vi "Spi Master.vi"(0 "spi input":T1, 5 "manual assert chip select":bool, 7 "start strobe":bool, 9 "data to write":u64 format="%.0x", 11 "MOSI output enable done":bool=TRUE, 13 "spi transfer settings":T2 {"Direction Change Bit" max=64 step=1; "Transfer Length (bits)" min=1 max=64 step=1}) -> (4 "spi output":T3, 8 "read data valid":bool, 10 "read data":u64 format="%.0x", 14 "ready for input":bool)   [LabVIEW 2014, in "NI SPI IP (FPGA).lvlib"]
doc: "This VI implements a SPI master that is compliant with both 4-wire (unidirectional input and output data) and 3-wire (bidirectional input/output data) SPI transfers. \n\nPlease see the documentation included with this example for details on how to include this VI into your application.\n\n\"Start strobe\" should be asserted only when \"data to write\" is valid. \"Data to write\" is latched when the start strobe asserts."
uses:
  <userlib>/_NI SPI IP/FPGA/Controllers/NI SPI IP (FPGA).lvlib
  <userlib>/_NI SPI IP/FPGA/Controllers/Public/Spi Master Outputs.ctl
  <userlib>/_NI SPI IP/FPGA/Controllers/Public/Transfer Settings.ctl
  <userlib>/_NI SPI IP/FPGA/Controllers/Public/Spi Master Inputs.ctl
  <userlib>/_NI SPI IP/FPGA/Controllers/Private/Master State.ctl
  <userlib>/_NI SPI IP/FPGA/Controllers/Private/Controller Interface.ctl
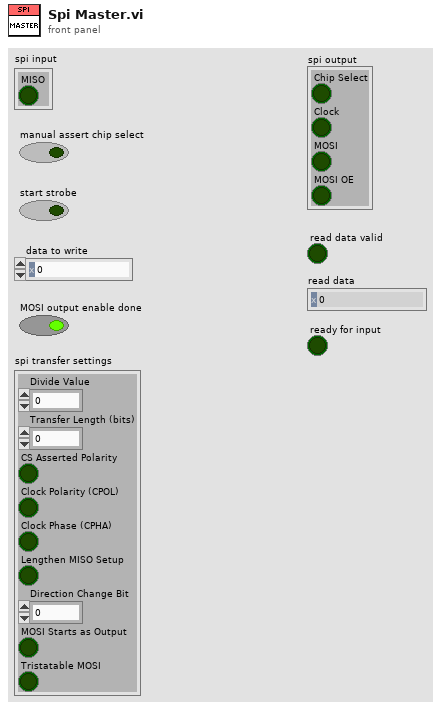
[diagram p1: front panel]
types:
  T1 = typedef "NI SPI IP (FPGA).lvlib/Spi Master Inputs.ctl" = cluster{"MISO":bool}
  T2 = typedef "NI SPI IP (FPGA).lvlib/Transfer Settings.ctl" = cluster{"Divide Value":u8, "Transfer Length (bits)":u8, "CS Asserted Polarity":bool, "Clock Polarity (CPOL)":bool, "Clock Phase (CPHA)":bool, "Lengthen MISO Setup":bool, "Direction Change Bit":u8, "MOSI Starts as Output":bool, "Tristatable MOSI":bool}
  T3 = typedef "NI SPI IP (FPGA).lvlib/Spi Master Outputs.ctl" = cluster{"Chip Select":bool, "Clock":bool, "MOSI":bool, "MOSI OE":bool}
  T4 = typedef "NI SPI IP (FPGA).lvlib/Controller Interface.ctl" = cluster{"Load":bool, "Divider Pulse":bool, "Enable Data":bool, "Clear Mosi":bool}
  T5 = typedef "NI SPI IP (FPGA).lvlib/Master State.ctl" = enum16{"Idle", "Load", "AssertChipSelect", "SendData", "DeassertChipSelect", "Done", "Change MOSI Direction", "WaitForDirChangeDone"}
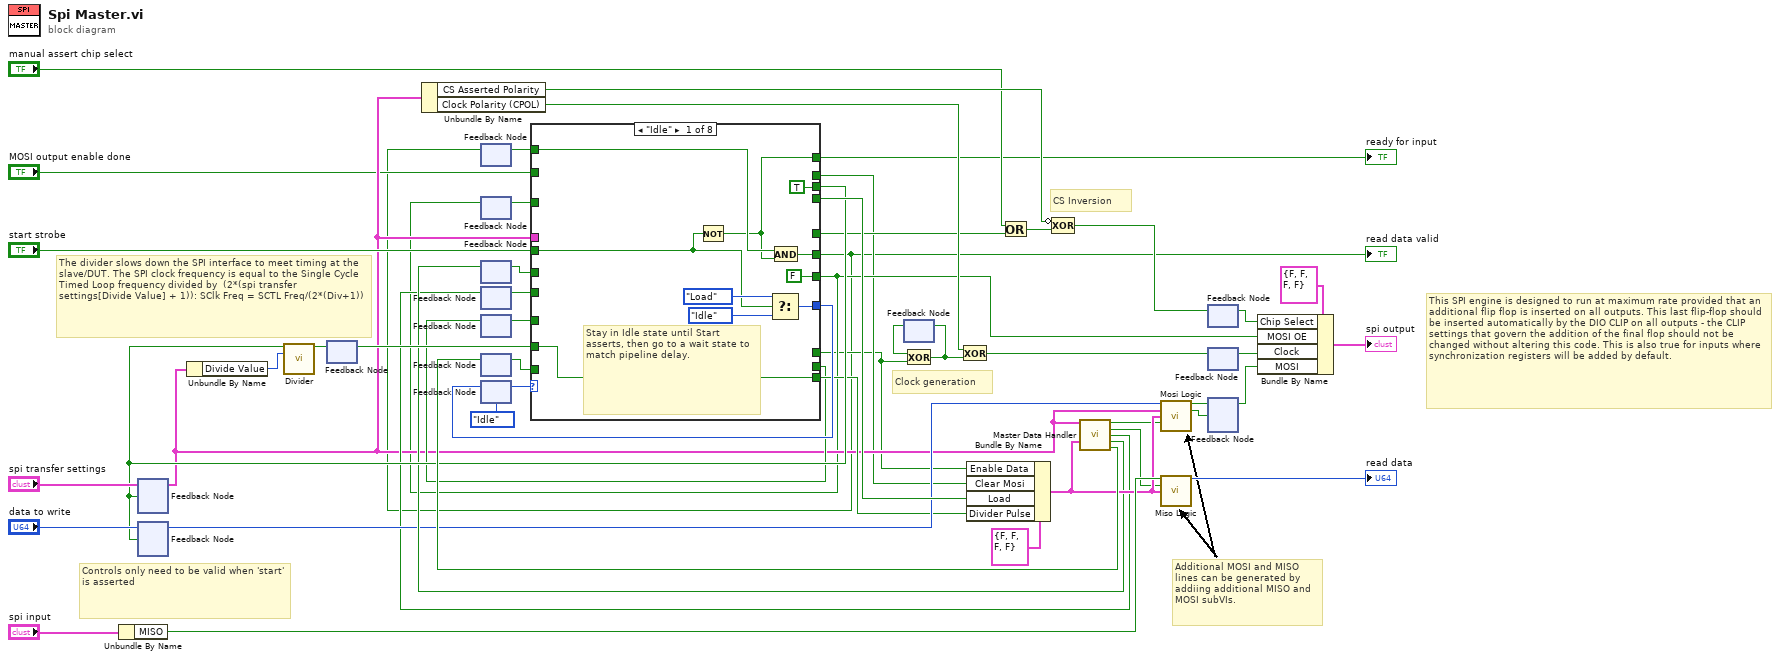
[diagram p0: block diagram]
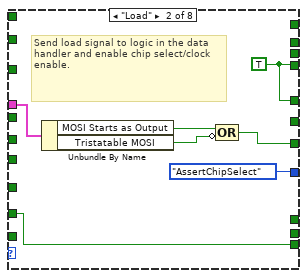
[diagram p2: hidden frame]
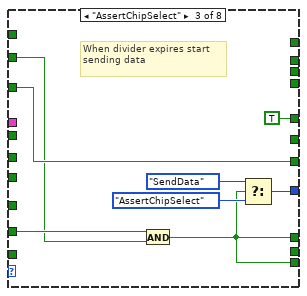
[diagram p3: hidden frame]
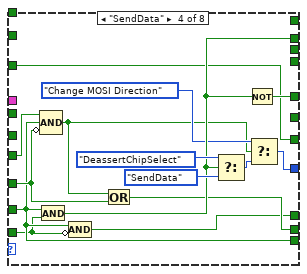
[diagram p4: hidden frame]
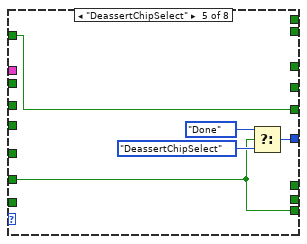
[diagram p5: hidden frame]
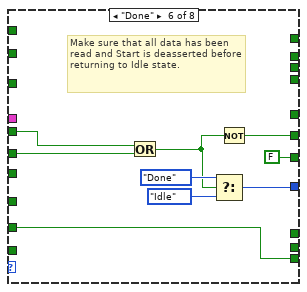
[diagram p6: hidden frame]
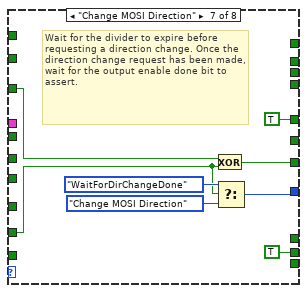
[diagram p7: hidden frame]
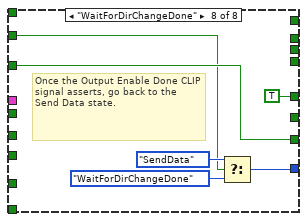
[diagram p8: hidden frame]
diagram:
  # "CS Inversion"
  # "Additional MOSI and MISO lines can be generated by addiing additional MISO and MOSI subVIs."
  # "Controls only need to be valid when 'start' is asserted"
  # "Clock generation"
  # "This SPI engine is designed to run at maximum rate provided that an additional flip flop is inserted on all outputs. This last flip-flop should be inserted automatically by the DIO CLIP on all outputs - the CLIP settings that govern the addition of the final flop should not be changed without altering this code. This is also true for inputs where synchronization registers will be added by default."
  # "The divider slows down the SPI interface to meet timing at the slave/DUT. The SPI clock frequency is equal to the Single Cycle Timed Loop frequency divided by  (2*(spi transfer settings[Divide Value] + 1)): SClk Freq = SCTL Freq/(2*(Div+1))"
  n1 = Unbundle By Name("spi input") -> ("MISO"=w29:bool)
  n2 = feedback #1() -> (w11:T2)  [unwired: 1 in]
  n3 = feedback #2() -> (w23:u64)  [unwired: 1 in]
  n4 = Unbundle By Name(w11) -> ("Divide Value"=w49:u8)
  n5 = feedback #3() -> (w35:bool)  [unwired: 1 in]
  n6 = Unbundle By Name(w11) -> ("CS Asserted Polarity"=w31:bool, "Clock Polarity (CPOL)"=w46:bool)
  n7 = feedback #4() -> (w1:bool)  [unwired: 1 in]
  n8 = feedback #5() -> (w16:bool)  [unwired: 1 in]
  n9 = feedback #6() -> (w39:bool)  [unwired: 1 in]
  n10 = feedback #7() -> (w17:bool)  [unwired: 1 in]
  n11 = feedback #8() -> (w13:bool)  [unwired: 1 in]
  n12 = feedback #9() -> (w47:bool)  [unwired: 1 in]
  n13 = feedback #10(Master_State."Idle" ("Enum")) -> (w51:T5)
  n14 = case shown="\"Idle\"" w51 {
    tunnel: [w63 Master_State."AssertChipSelect" ("Enum") w76 w88 w97 w107 w114 w118] -> w52
    tunnel: w35 -> [w59 w68 w73 w83 w94 w102 w108 _]
    tunnel: [w56 _ _ _ _ _ _ _] -> w3
    tunnel: "start strobe" -> [w55 _ _ _ _ w104 _ _]
    tunnel: [_ w69 TRUE w91 _ _ TRUE ("Clock") TRUE ("Clock")] -> w20
    tunnel: w47 -> [_ _ _ w82 _ _ _ _]
    tunnel: [_ _ w71 w81 _ _ _ _] -> w4
    tunnel: [_ w69 _ _ _ _ _ _] -> w44
    tunnel: [TRUE ("Clock") _ _ _ _ _ _ _] -> w27
    tunnel: [_ _ _ w90 _ _ _ _] -> w5
    tunnel: w39 -> [_ _ _ _ _ w103 _ _]
    tunnel: w17 -> [_ _ _ w79 _ _ _ _]
    tunnel: [FALSE w64 w74 w80 w95 FALSE w109 w119] -> w6
    tunnel: w16 -> [_ _ w74 w80 w95 _ w110 w119]
    tunnel: [w59 w68 w71 w83 w94 w102 _ _] -> w15
    tunnel: [_ _ _ w84 _ _ TRUE _] -> w14
    tunnel: w13 -> [_ _ _ w85 _ _ _ _]
    tunnel: w11 -> [_ w67 _ _ _ _ _ _]
    tunnel: "MOSI output enable done" -> [_ _ w72 _ _ _ _ w116]
    tunnel: [w58 _ _ _ _ w100 _ _] -> w2
    tunnel: w1 -> [w57 _ _ _ _ _ _ _]
    frame "Idle" {
      # "Stay in Idle state until Start asserts, then go to a wait state to match pipeline delay."
      n15 = Not(x=w55) -> (.not. x?=w56:bool)
      n16 = Select(t=Master_State."Load" ("Enum"), s=w55, f=Master_State."Idle" ("Enum")) -> (s? t:f=w63:T5)
      n17 = And(x=w57, y=w56) -> (x .and. y?=w58:bool)
    }
    frame "Load" {
      w69 = TRUE ("Clock")
      # "Send load signal to logic in the data handler and enable chip select/clock enable."
      n18 = Unbundle By Name(w67) -> ("MOSI Starts as Output"=w66:bool, "Tristatable MOSI"=w65:bool)
      n19 = Compound Arithmetic op=OR(w66, invert w65) -> (w64:bool)
    }
    frame "AssertChipSelect" {
      # "When divider expires start sending data"
      n20 = And(x=w73, y=w72) -> (x .and. y?=w71:bool)
      n21 = Select(t=Master_State."SendData" ("Enum"), s=w71, f=Master_State."AssertChipSelect" ("Enum")) -> (s? t:f=w76:T5)
    }
    frame "SendData" {
      n22 = And(x=w83, y=w82) -> (x .and. y?=w90:bool)
      n23 = Compound Arithmetic op=AND(w79, w83, invert w85) -> (w86:bool)
      n24 = Compound Arithmetic op=AND(w83, invert w82) -> (w81:bool)
      n25 = Or(x=w86, y=w85) -> (x .or. y?=w84:bool)
      n26 = Select(t=Master_State."DeassertChipSelect" ("Enum"), s=w90, f=Master_State."SendData" ("Enum")) -> (s? t:f=w89:T5)
      n27 = Not(x=w90) -> (.not. x?=w91:bool)
      n28 = Select(t=Master_State."Change MOSI Direction", s=w86, f=w89) -> (s? t:f=w88:T5)
    }
    frame "DeassertChipSelect" {
      n29 = Select(t=Master_State."Done" ("Enum"), s=w94, f=Master_State."DeassertChipSelect" ("Enum")) -> (s? t:f=w97:T5)
    }
    frame "Done" {
      # "Make sure that all data has been read and Start is deasserted before returning to Idle state."
      n30 = Or(x=w104, y=w103) -> (x .or. y?=w101:bool)
      n31 = Select(t=Master_State."Done" ("Enum"), s=w101, f=Master_State."Idle" ("Enum")) -> (s? t:f=w107:T5)
      n32 = Not(x=w101) -> (.not. x?=w100:bool)
    }
    frame "Change MOSI Direction" {
      # "Wait for the divider to expire before requesting a direction change. Once the direction change request has been made, wait for the output enable done bit to assert."
      n33 = Exclusive Or(1:w108, 2:w110) -> (0:w109:bool)
      n34 = Select(t=Master_State."WaitForDirChangeDone" ("Enum"), s=w108, f=Master_State."Change MOSI Direction" ("Enum")) -> (s? t:f=w114:T5)
    }
    frame "WaitForDirChangeDone" {
      # "Once the Output Enable Done CLIP signal asserts, go back to the Send Data state."
      n35 = Select(t=Master_State."SendData" ("Enum"), s=w116, f=Master_State."WaitForDirChangeDone" ("Enum")) -> (s? t:f=w118:T5)
    }
  }
  "ready for input" <- w3
  "read data valid" <- w2
  n36 = feedback-in #1("spi transfer settings", w27) -> ()
  n37 = feedback-in #2("data to write", w27) -> ()
  n38 = call <userlib>:"Divider.vi"("reset"=w27, "divide value"=w49) -> ("count done"=w48:bool)  [unwired: 13 in]
  n39 = feedback-in #3(w48) -> ()
  n40 = feedback-in #4(w2) -> ()
  n41 = feedback-in #5(w6) -> ()
  n42 = feedback-in #8(w14) -> ()
  n43 = feedback-in #10(w52) -> ()
  n44 = feedback #11() -> (w42:bool)  [unwired: 1 in]
  n45 = Exclusive Or(1:w4, 2:w42) -> (0:w18:bool)
  n46 = feedback-in #11(w18) -> ()
  n47 = Exclusive Or(1:w18, 2:w46) -> (0:w45:bool)
  n48 = Bundle By Name(cluster=T4 {"Load"=FALSE, "Divider Pulse"=FALSE, "Enable Data"=FALSE, "Clear Mosi"=FALSE} ("ControllerInterface"), "Enable Data"=w4, "Clear Mosi"=w5, "Load"=w44, "Divider Pulse"=w15) -> (w28:T4)
  n49 = Or(x="manual assert chip select", y=w20) -> (x .or. y?=w9:bool)
  n50 = Compound Arithmetic op=XOR(invert w31, w9) -> (w41:bool)
  n51 = call <userlib>:"Master Data Handler.vi"("transfer settings"=w11, "controller interface"=w28) -> ("shift MOSI"=w25:bool, "sample MISO"=w24:bool, "dir change"=w12:bool, "read pending"=w26:bool, "done"=w43:bool)  [unwired: 9 in]
  n52 = feedback-in #6(w26) -> ()
  n53 = feedback-in #7(w12) -> ()
  n54 = feedback-in #9(w43) -> ()
  n55 = call <userlib>:"Mosi Logic.vi"("data to send"=w23, "transfer settings"=w11, "controller interface"=w28, "shift MOSI"=w25) -> ("MOSI"=w22:bool, "MOSI enable"=w21:bool)  [unwired: 10 in]
  n56 = call <userlib>:"Miso Logic.vi"("MISO"=w29, "sample MISO"=w24, "controller interface"=w28) -> ("read data"=→"read data":u64)  [unwired: 12 in]
  n57 = feedback #12() -> (w40:bool)  [unwired: 1 in]
  n58 = feedback-in #12(w41) -> ()
  n59 = feedback #13() -> (w7:bool)  [unwired: 1 in]
  n60 = feedback-in #13(w45) -> ()
  n61 = feedback #14() -> (w8:bool)  [unwired: 1 in]
  n62 = feedback-in #14(w22, w21) -> ()
  n63 = Bundle By Name(cluster=T3 {"Chip Select"=FALSE, "Clock"=FALSE, "MOSI"=FALSE, "MOSI OE"=FALSE} ("SPI.Output"), "Chip Select"=w40, "MOSI OE"=w6, "Clock"=w7, "MOSI"=w8) -> (→"spi output":T3)
